vi "Timing Test.vi"() -> ()   [LabVIEW 2025]
panel:
  out "Time Left (s)":dbl
  out "Time Left (ms)":i32
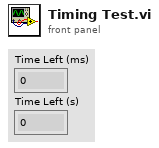
[diagram p1: front panel]
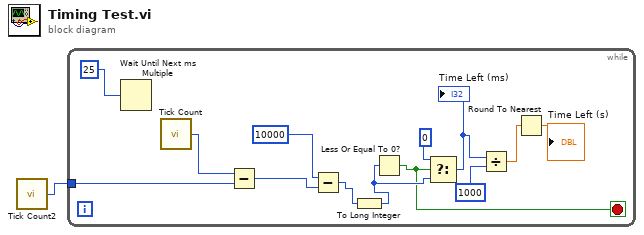
[diagram p0: block diagram]
diagram:
  n1 = call "Tick Count2"() -> ("Tick Count(mSec)"=w1:u32)
  n2 = while {
    tunnel: w1 -> [w14]
    stop <- w4 stop-if-true
    n3 = Wait Until Next ms Multiple(millisecond multiple=u32 25) -> ()  [unwired: 1 out]
    n4 = call "Tick Count"() -> ("Tick Count(mSec)"=w13:u32)
    n5 = Subtract(x=w13, y=w14) -> (x-y=w11:u32)
    n6 = Subtract(x=u32 10000, y=w11) -> (x-y=w9:u32)
    n7 = To Long Integer(number=w9) -> (32bit integer=w7:i32)
    n8 = Less Or Equal To 0?(x=w7) -> (x <= 0?=w4:bool)
    n9 = Select(t=0, s=w4, f=w7) -> (s? t:f=w6:i32)
    "Time Left (ms)" <- w6
    n10 = Divide(x=w6, y=1000) -> (x/y=w3:dbl)
    n11 = Round To Nearest(number=w3) -> (nearest integer value=→"Time Left (s)":dbl)
  }
